vi "Diagnosewerte loggen.vi"(8 "error in (no error)":errorcluster caption="Fehler (Eingang, kein Fehler)") -> (0 "error out":errorcluster caption="Fehler (Ausgang)")   [LabVIEW 2020, in "FT-IR.lvlib"]
uses:
  FT-IR.lvlib
  FGV FT-IR Diagnose Aktionen.ctl
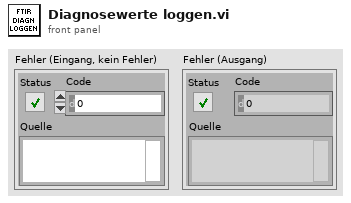
[diagram p1: front panel]
types:
  T1 = typedef "FT-IR.lvlib/FGV FT-IR Diagnose Aktionen.ctl" = enum16{"Lesen", "Diagnose Schreiben", "Min Schreiben", "Max Schreiben"}
  T2 = enum16{"open", "replace", "create", "open or create", "replace or create", "replace or create with confirmation"}
  T3 = typedef "FT-IR.lvlib/TOOLweb Interface.lvlib/Typdefinitionen.lvlib/TOOLweb Diagnose.ctl" = cluster{"(14) temperature":sgl, "(15) pressure":sgl, "(16) oxygen":sgl, "(50) diag-igramdc":sgl, "(51) diag-igrampp":sgl, "(52) diag-phaseAngle":sgl, "(53) diag-laserpp":sgl, "(54) diag-laserdc":sgl, "(55) diag-badscan":sgl, "(56) diag-centerburst":sgl, "(57) diag-linearizerCheck":sgl, "(58) diag-SNR":sgl, "(59) diag-sBeamIntensity":sgl}
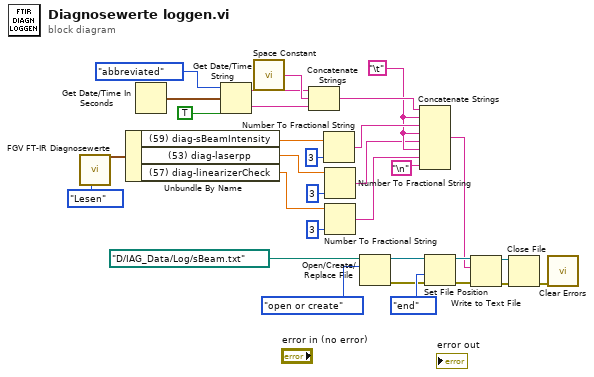
[diagram p0: block diagram]
diagram:
  w4 = "\t"
  n1 = call "FGV FT-IR Diagnosewerte.vi"("Aktionen"=FGV_FT-IR_Diagnose_Aktionen."Lesen") -> ("Diagnose"=w20:T3)  [unwired: 5 in, 5 out]
  n2 = Unbundle By Name(w20) -> ("(59) diag-sBeamIntensity"=w13:sgl, "(53) diag-laserpp"=w5:sgl, "(57) diag-linearizerCheck"=w6:sgl)
  n3 = Get Date/Time In Seconds() -> (seconds since 1Jan1904=w14:timestamp)
  n4 = Get Date/Time String(date format (0)=enum16{"short", "long", "abbreviated"}."abbreviated" ("Datumsformat (0)"), seconds (now)=w14, want seconds? (F)=TRUE ("Angabe von Sekunden? (F)")) -> (date string=w17:string, time string=w19:string)
  n5 = call <vilib>:"Space Constant.vi"() -> ("String"=w18:string)
  n6 = Concatenate Strings(w17, w18, w19) -> (w11:string)
  n7 = Number To Fractional String(number=w13, precision (6)=i16 3 ("Breite (-)")) -> (F-format string=w10:string)  [unwired: 2 in]
  n8 = Number To Fractional String(number=w5, precision (6)=i16 3 ("Breite (-)")) -> (F-format string=w3:string)  [unwired: 2 in]
  n9 = Number To Fractional String(number=w6, precision (6)=i16 3 ("Breite (-)")) -> (F-format string=w2:string)  [unwired: 2 in]
  n10 = Open/Create/Replace File(file path (use dialog)=path "D:/IAG_Data/Log/sBeam.txt" ("Dateipfad (Dialog verwenden)"), operation (0:open)=T2."open or create" ("Operation (0:Öffnen)")) -> (refnum out=w25:refnum<file>, error out=w26:errorcluster)  [unwired: 4 in, 1 out]
  n11 = Concatenate Strings(w11, w4, w10, w4, w3, w4, w2, "\n") -> (w12:string)
  n12 = Set File Position(refnum=w25, from (0:start)=enum16{"start", "end", "current"}."end" ("Von (0:Start)"), error in=w26) -> (refnum out=w24:refnum<file>, error out=w23:errorcluster)  [unwired: 1 in]
  n13 = Write to Text File(file (use dialog)=w24, text=w12, error in=w23) -> (refnum out=w30:refnum<file>, error out=w31:errorcluster)  [unwired: 1 in, 1 out]
  n14 = Close File(refnum=w30, error in=w31) -> (error out=w29:errorcluster)  [unwired: 1 out]
  n15 = call <vilib>:"Clear Errors.vi"("error in (no error)"=w29) -> ()  [unwired: 5 in, 2 out]
